vi "JSON to LVObject.vi"(7 "JSONtext LVClass Serializer in":refnum<class "JSONtext LVClass Serializer.lvclass">, 8 "error in (no error)":errorcluster, 9 "Object Type":refnum<class>, 10 "Offset":i32, 11 "JSON":string) -> (0 "error out":errorcluster, 1 "Object":refnum<class>)   [LabVIEW 2019, in "JSONtext LVClass Serializer.lvclass"]
doc: "Convert JSON to an Object of a LabVIEW Class."
uses:
  JSONtext LVClass Serializer.lvclass
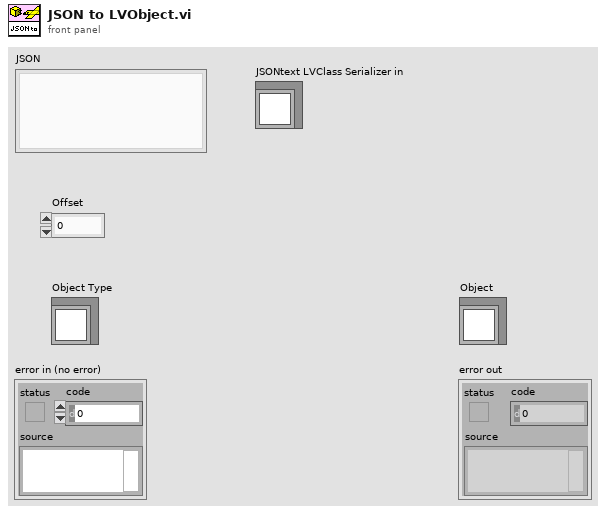
[diagram p1: front panel]
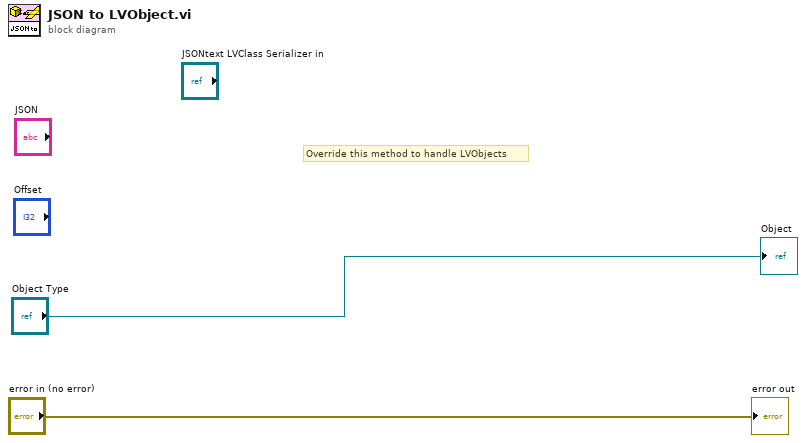
[diagram p0: block diagram]
diagram:
  # "Override this method to handle LVObjects"
  "error out" <- "error in (no error)"
  "Object" <- "Object Type"
